vi "Andor_iXon_Average_Picture_Intensity.vi"(8 "Input Cluster":T6) -> (0 "Numeric":dbl)   [LabVIEW 2009]
uses:
  atmcd32d.llb/AcquisitionMode_mode typedef.ctl
  atmcd32d.llb/ReadMode_mode typedef.ctl
  atmcd32d.llb/TriggerMode_mode typedef.ctl
  atmcd32d.llb/Shutter_type typedef.ctl
  atmcd32d.llb/Shutter_mode typedef.ctl
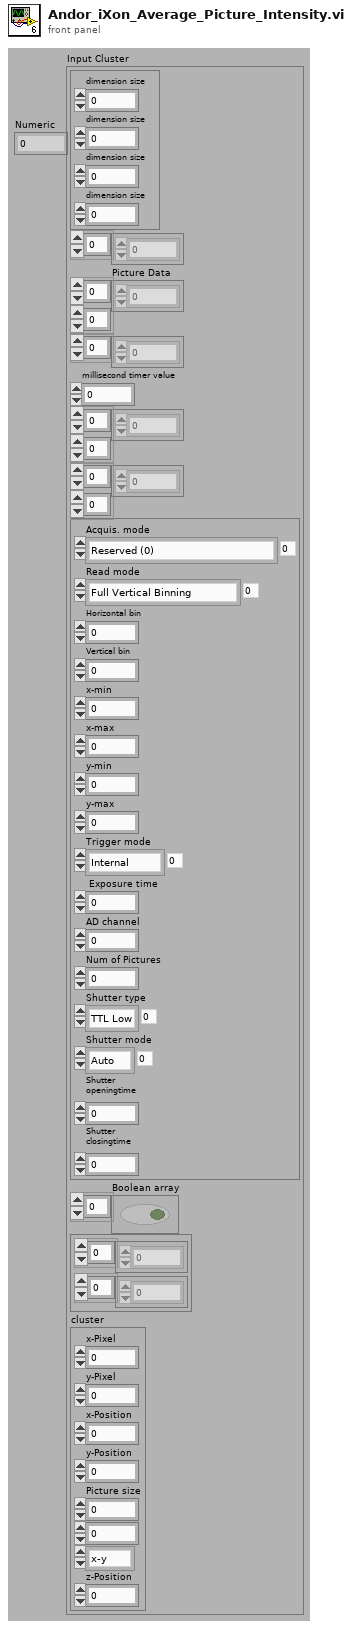
[diagram p1: front panel]
types:
  T1 = typedef "AcquisitionMode_mode typedef.ctl" = enum16{"Reserved (0)", "Single Scan", "Accumulate", "Kinetics", "Fast Kinetics", "Run Till Abort", "Reserved (6)", "Reserved (7)", "Reserved (8)", "Time Delayed Integration"}
  T2 = typedef "ReadMode_mode typedef.ctl" = enum16{"Full Vertical Binning", "Multi-Track", "Random-Track", "Single-Track", "Image"}
  T3 = typedef "TriggerMode_mode typedef.ctl" = enum16{"Internal", "External", "N/A (2)", "N/A (3)", "N/A (4)", "N/A (5)", "External Start"}
  T4 = typedef "Shutter_type typedef.ctl" = enum16{"TTL Low", "TTL High"}
  T5 = typedef "Shutter_mode typedef.ctl" = enum16{"Auto", "Open", "Close"}
  T6 = cluster{cluster{"dimension size":i32, "dimension size":i32, "dimension size":i32, "dimension size":i32}, i32[], "Picture Data":dbl[][], u32[], "millisecond timer value":u32, dbl[][], i32[][], cluster{"Acquis. mode":T1, "Read mode":T2, "Horizontal bin":i32, "Vertical bin":i32, "x-min":i32, "x-max":i32, "y-min":i32, "y-max":i32, "Trigger mode":T3, " Exposure time":sgl, "AD channel":i32, "Num of Pictures":i32, "Shutter type":T4, "Shutter mode":T5, "Shutter\nopeningtime":i32, "Shutter\nclosingtime":i32}, "Boolean array":bool[], cluster{dbl[], dbl[]}, "cluster":cluster{"x-Pixel":u16, "y-Pixel":u16, "x-Position":dbl, "y-Position":dbl, "Picture size":dbl, dbl, enum32{"x-y", "x-z", "y-z"}, "z-Position":dbl}}
  T7 = cluster{"dimension size":i32, "dimension size":i32, "dimension size":i32, "dimension size":i32}
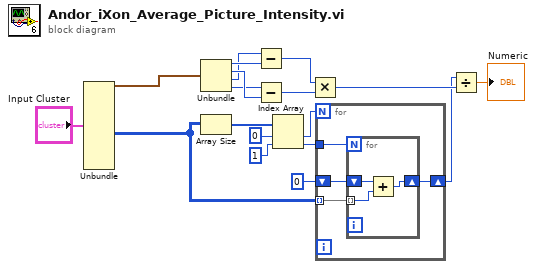
[diagram p0: block diagram]
diagram:
  n1 = Unbundle("Input Cluster") -> (w18:T7, w17:i32[][])  [unwired: 9 out]
  n2 = Unbundle(w18) -> ("dimension size"=w9:i32, "dimension size"=w11:i32, "dimension size"=w8:i32, "dimension size"=w10:i32)
  n3 = Array Size(array=w17) -> (size(s)=w2:i32[])
  n4 = Subtract(x=w8, y=w9) -> (x-y=w12:i32)
  n5 = Subtract(x=w10, y=w11) -> (x-y=w13:i32)
  n6 = Index Array(array=w2, index #1=0 ("index"), index #2=1 ("index")) -> (element #1=w5:i32, element #2=w6:i32)
  n7 = Multiply(x=w12, y=w13) -> (x*y=w15:i32)
  n8 = for {
    N: w5 -> [_]
    tunnel: w17 -> [w22] mode=indexing
    tunnel: w6 -> [w21]
    shift-right: [w19] -> w14
    shift-left: 0 ("index") -> [w20]
    n9 = for {
      N: w21 -> [_]
      tunnel: w22 -> [w24] mode=indexing
      shift-right: [w23] -> w19
      shift-left: w20 -> [w25]
      n10 = Add(x=w25, y=w24) -> (x+y=w23:i32)
    }
  }
  n11 = Divide(x=w14, y=w15) -> (x/y=→"Numeric":dbl)
